vi "TBA_NET_Click Call Back.vi"(4 "ToolbarClick":refnum<user-event>, 5 "事件数据":cluster{"sender":refnum<k24>, "e":refnum<k24>}, 6 "控件引用":refnum<k24>, 7 "事件通用数据":cluster{"事件源":i32, "事件类型":u32, "时间标识":u32}) -> ()   [LabVIEW 2016]
uses:
  System.Windows.Forms
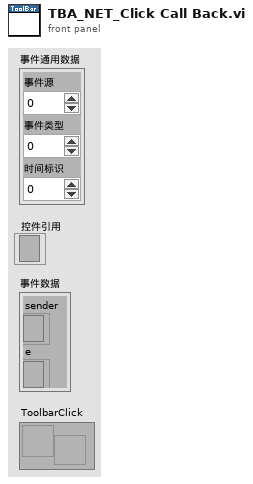
[diagram p1: front panel]
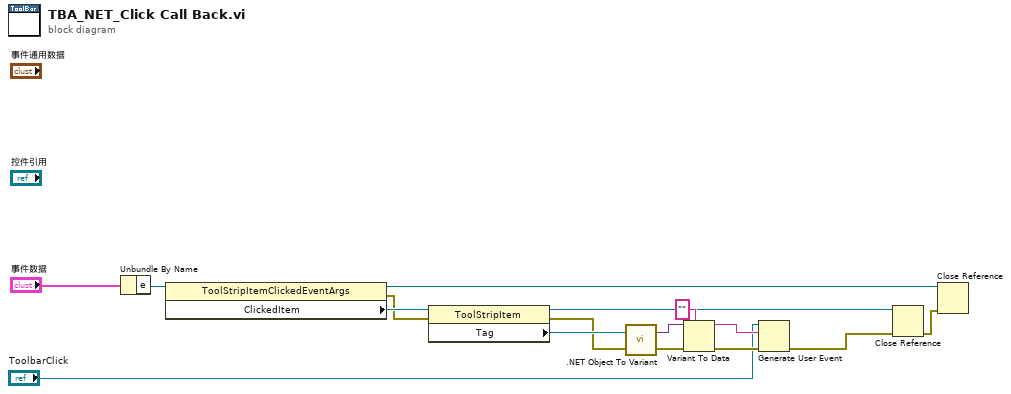
[diagram p0: block diagram]
diagram:
  n1 = Unbundle By Name("事件数据") -> ("e"=w13:refnum<k24>)
  n2 = property class="ToolStripItemClickedEventArgs"(reference=w13) -> (reference out=w4:refnum<k24>, error out=w11:errorcluster, "ClickedItem"=w12:refnum<k24>)  [unwired: 1 in]
  n3 = property class="ToolStripItem"(reference=w12, error in=w11) -> (reference out=w6:refnum<k24>, error out=w9:errorcluster, "Tag"=w10:refnum<k24>)
  n4 = call <vilib>:".NET Object To Variant.vi"("error in (no error)"=w9, ".NET object"=w10) -> ("error out"=w16:errorcluster, "variant"=w15:variant)
  n5 = Variant To Data(error in=w16, type="", Variant=w15) -> (data=w8:string, error out=w7:errorcluster)
  n6 = Generate User Event(user event="ToolbarClick", event data cluster=w8, error in=w7) -> (error out=w2:errorcluster)  [unwired: 1 in, 1 out]
  n7 = Close Reference(reference=w6, error in (no error)=w2) -> (error out=w5:errorcluster)
  n8 = Close Reference(reference=w4, error in (no error)=w5) -> ()  [unwired: 1 out]
